vi "Add Slave Test Runner.vi"(8 "error in (no error)":errorcluster, 11 "Test Runner in":refnum<class "Test Runner.lvclass">) -> (0 "error out":errorcluster, 3 "Test Runner out":refnum<class "Test Runner.lvclass">)   [LabVIEW 2020, in "Test Runner.lvclass"]
uses:
  Test Runner.lvclass
  C:/Git/astemes-lunit/source/Application Framework/Process Classes/Process/Process.lvclass
  Application Framework/Process Classes/Process/Process.lvclass/Process.ctl
  Slave Test Runner/Slave Test Runner.lvclass
  Test Runner.lvclass/Test Runner.ctl
  Slave Test Runner/Slave Test Runner.lvclass/Slave Test Runner.ctl
  Application Framework/Process Classes/Process/Protected/Messaging/Enqueue Message.vi
  Application Framework/Process Classes/Process/Process.lvclass
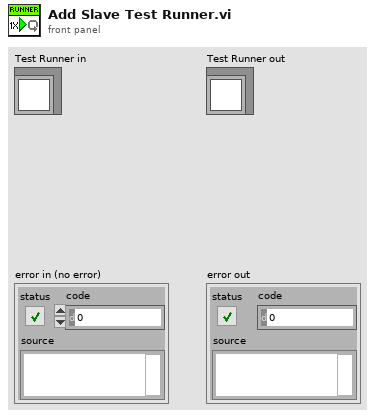
[diagram p1: front panel]
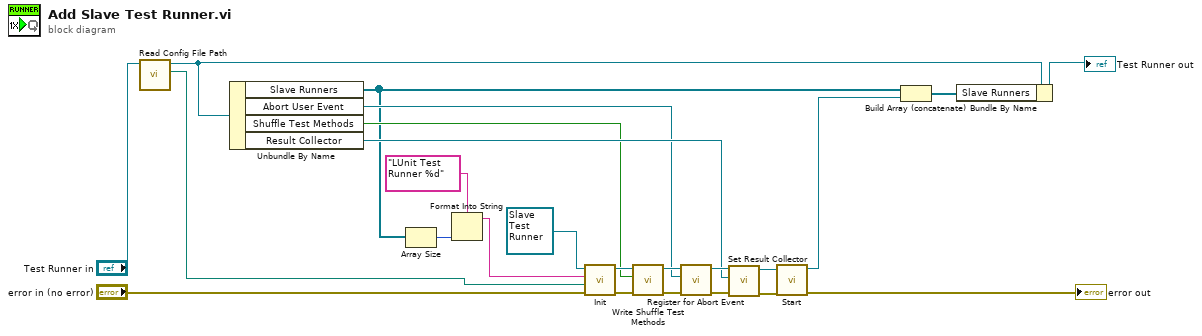
[diagram p0: block diagram]
diagram:
  n1 = call "Read Config File Path.vi"("Process In"="Test Runner in") -> ("Config File Path"=w14:path, "Process Out"=w11:refnum<class "Test Runner.lvclass">)  [unwired: 9 in]
  n2 = Unbundle By Name(w11) -> ("Slave Runners"=w4:refnum<class "Slave Test Runner.lvclass">[], "Abort User Event"=w10:refnum<user-event>, "Shuffle Test Methods"=w13:bool, "Result Collector"=w15:refnum<class "Result Collector.lvclass">)
  n3 = Array Size(array=w4) -> (size(s)=w3:i32)
  n4 = Format Into String(format string="LUnit Test Runner %d", w3) -> (resulting string=w2:string)  [unwired: 2 in, 1 out]
  n5 = call-dynamic "Init.vi"("error in (no error)"="error in (no error)", "Config File Path"=w14, "Name"=w2, "Slave Test Runner In"=refnum<class "Slave Test Runner.lvclass"> refnum ("Test Runner In")) -> ("error out"=w17:errorcluster, "Slave Test Runner Out"=w18:refnum<class "Slave Test Runner.lvclass">)  [unwired: 6 in]
  n6 = call "Write Shuffle Test Methods.vi"("error in (no error)"=w17, "Shuffle Test Methods"=w13, "Slave Test Runner In"=w18) -> ("error out"=w19:errorcluster, "Slave Test Runner Out"=w20:refnum<class "Slave Test Runner.lvclass">)  [unwired: 7 in]
  n7 = call "Register for Abort Event.vi"("error in (no error)"=w19, "Abort User Event"=w10, "Slave Test Runner In"=w20) -> ("error out"=w21:errorcluster, "Slave Test Runner Out"=w23:refnum<class "Slave Test Runner.lvclass">)  [unwired: 7 in]
  n8 = call "Set Result Collector.vi"("error in (no error)"=w21, "Test Suite"=w15, "Slave Test Runner In"=w23) -> ("error out"=w22:errorcluster, "Slave Test Runner Out"=w24:refnum<class "Slave Test Runner.lvclass">)  [unwired: 7 in]
  n9 = call "Start.vi"("error in (no error)"=w22, "Process In"=w24) -> ("error out"=→"error out":errorcluster, "Process Out"=w5:refnum<class "Slave Test Runner.lvclass">)  [unwired: 8 in]
  n10 = Build Array (concatenate)(w4, w5) -> (w6:refnum<class "Slave Test Runner.lvclass">[])
  n11 = Bundle By Name(cluster=w11, "Slave Runners"=w6) -> (→"Test Runner out":refnum<class "Test Runner.lvclass">)
